vi "Read Assert Name List.vi"(11 "Base Display Configuration in":refnum<class "Base Display Configuration.lvclass">) -> (2 "Assert Name List":variant)   [LabVIEW 2016, in "Assert API Components.lvlib" / "Assert Display.lvlib" / "Main Display.lvlib" / "Base Display Configuration.lvclass"]
uses:
  Base Display Configuration.lvclass
  Base Display Configuration.lvclass/Base Display Configuration.ctl
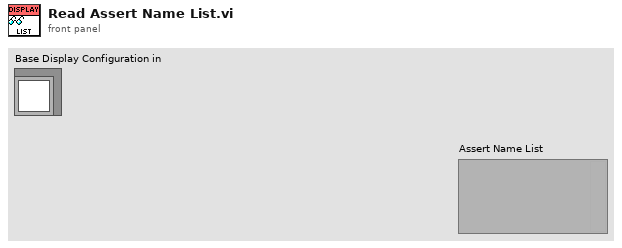
[diagram p1: front panel]
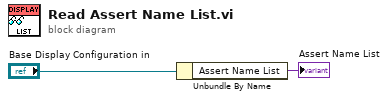
[diagram p0: block diagram]
diagram:
  n1 = Unbundle By Name("Base Display Configuration in") -> ("Assert Name List"=→"Assert Name List":variant)
